vi "Unflatten.vi"(8 "error in (no error)":errorcluster, 11 "Magnetic Field in":refnum<class "Magnetic Field Oxford.lvclass">) -> (0 "error out":errorcluster, 3 "Magnetic Field out":refnum<class "Magnetic Field Oxford.lvclass">)   [LabVIEW 2017, in "Magnetic Field Oxford.lvclass"]
uses:
  Magnetic Field Oxford.lvclass
  Magnetic Field Oxford.lvclass/Magnetic Field Oxford.ctl
  Global/File Locations.vi
  Scanner/Scanner.lvclass
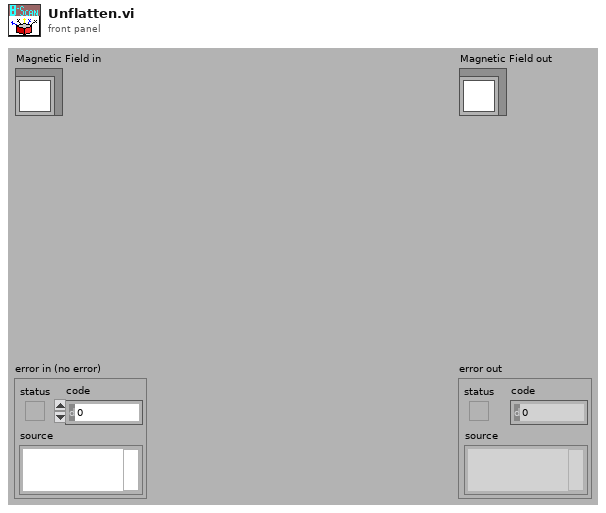
[diagram p1: front panel]
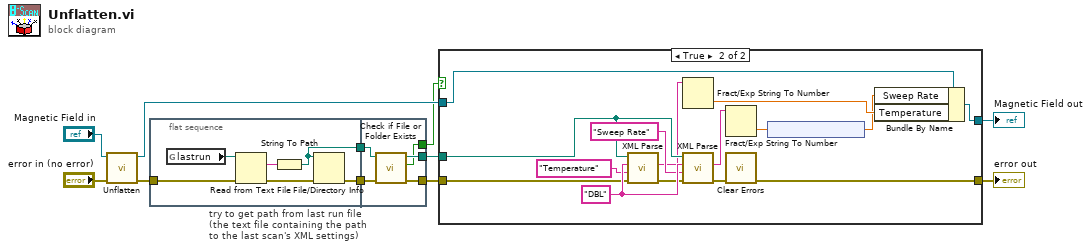
[diagram p0: block diagram]
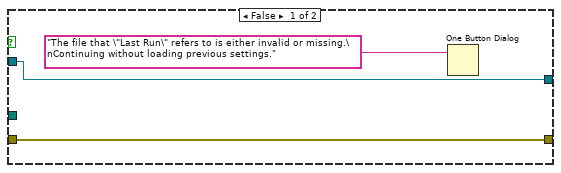
[diagram p2: hidden frame]
diagram:
  n1 = call-parent "Unflatten.vi"("error in (no error)"="error in (no error)", "Scanner in"="Magnetic Field in") -> ("error out"=w5:errorcluster, "Scanner out"=w11:refnum<class "Magnetic Field Oxford.lvclass">)  [unwired: 8 in]
  n2 = flat-sequence "try to get path from last run file\n(the text file containing the path\nto the last scan's XML settings)" {
    tunnel: w5 -> [w12]
    tunnel: [w17] -> w4
    tunnel: [w13] -> w3
    tunnel: [w20] -> w6
    tunnel: [w19] -> w7
    tunnel: w4 -> [w22]
    tunnel: w3 -> [w21]
    tunnel: [w18] -> w1
    frame #0 {
      n3 = global read "File Locations.vi" "lastrun"() -> (w15:path)
      n4 = Read from Text File(file (use dialog)=w15, error in=w12) -> (text=w16:string, error out=w14:errorcluster)  [unwired: 4 out]
      n5 = String To Path(string=w16) -> (path=w17:path)
      n6 = File/Directory Info(path=w17, error in=w14) -> (error out=w13:errorcluster)  [unwired: 6 out]
    }
    frame #1 {
      n7 = call <vilib>:"Check if File or Folder Exists.vi"("error in (no error)"=w21, "path"=w22) -> ("error out"=w20:errorcluster, "file or folder exists?"=w18:bool, "dup path"=w19:path)  [unwired: 7 in]
    }
  }
  n8 = case shown="True" w1 {
    tunnel: w11 -> [w24 w40]
    tunnel: [w24 w39] -> w8
    tunnel: w7 -> [_ w38]
    tunnel: w6 -> [w23 w34]
    tunnel: [w23 w26] -> w2
    frame False {
      n9 = One Button Dialog(message="The file that \"Last Run\" refers to is either invalid or missing.\nContinuing without loading previous settings.") -> ()  [unwired: 1 in, 1 out]
    }
    frame True {
      w37 = "DBL"
      n10 = call "XML Parse.vi"("error in (no error)"=w34, "Name String"="Temperature", "Type String"=w37, "Path"=w38) -> ("error out"=w33:errorcluster, "String Out"=w32:string)  [unwired: 6 in]
      n11 = Fract/Exp String To Number(string=w32) -> (number=w29:dbl)  [unwired: 3 in, 1 out]
      n12 = call "XML Parse.vi"("error in (no error)"=w33, "Name String"="Sweep Rate", "Type String"=w37, "Path"=w38) -> ("error out"=w27:errorcluster, "String Out"=w31:string)  [unwired: 6 in]
      n13 = Fract/Exp String To Number(string=w31) -> (number=w30:dbl)  [unwired: 3 in, 1 out]
      n14 = call <vilib>:"Clear Errors.vi"("error in (no error)"=w27) -> ("error out"=w26:errorcluster)  [unwired: 5 in, 1 out]
      n15 = node(w30) -> (w28:dbl[unit])
      n16 = Bundle By Name(cluster=w40, "Sweep Rate"=w28, "Temperature"=w29) -> (w39:refnum<class "Magnetic Field Oxford.lvclass">)
    }
  }
  "Magnetic Field out" <- w8
  "error out" <- w2
